vi "Bearing to graph.vi"(10 "Bearing":dbl=0.1) -> (2 "XY Graph":cluster{dbl[], dbl[]}(graph))   [LabVIEW 2009]
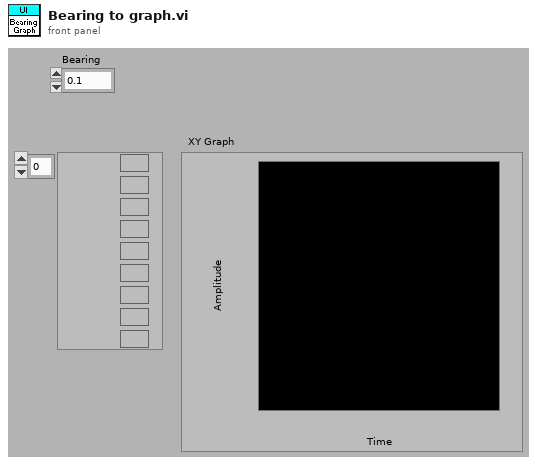
[diagram p1: front panel]
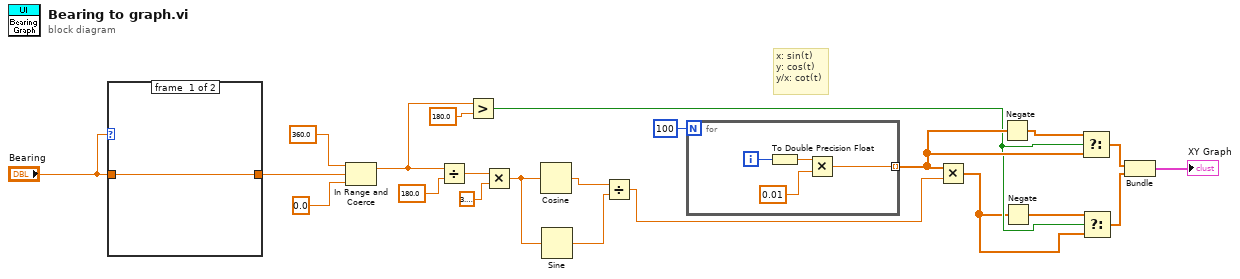
[diagram p0: block diagram]
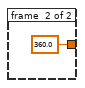
[diagram p2: hidden frame]
diagram:
  # "x: sin(t)\ny: cos(t)\ny/x: cot(t)"
  n1 = case shown="Default" "Bearing" {
    tunnel: [w23 360.0 ("Bearing")] -> w14
    tunnel: "Bearing" -> [w23 _]
    frame #0 {
    }
    frame #1 {
    }
  }
  n2 = In Range and Coerce(upper limit=360.0, x=w14, lower limit=0.0) -> (coerced(x)=w11:dbl)  [unwired: 1 out]
  n3 = Divide(x=w11, y=180.0) -> (x/y=w20:dbl)
  n4 = Greater?(x=w11, y=180.0) -> (0:w5:bool)
  n5 = Multiply(x=w20, y=3.141592653589793) -> (x*y=w18:dbl)
  n6 = Cosine(x=w18) -> (cos(x)=w16:dbl)
  n7 = Sine(x=w18) -> (sin(x)=w15:dbl)
  n8 = Divide(x=w16, y=w15) -> (x/y=w17:dbl)
  n9 = for {
    N: 100 -> [_]
    tunnel: [w25] -> w8 mode=indexing
    i -> [w28]
    n10 = To Double Precision Float(number=w28) -> (double precision float=w27:dbl)
    n11 = Multiply(x=w27, y=0.01) -> (x*y=w25:dbl)
  }
  n12 = Multiply(x=w8, y=w17) -> (x*y=w4:dbl[])
  n13 = Negate(x=w8) -> (-x=w9:dbl[])
  n14 = Negate(x=w4) -> (-x=w6:dbl[])
  n15 = Select(t=w9, s=w5, f=w8) -> (s? t:f=w7:dbl[])
  n16 = Select(t=w6, s=w5, f=w4) -> (s? t:f=w3:dbl[])
  n17 = Bundle(w7, w3) -> (→"XY Graph":cluster{dbl[], dbl[]})  [unwired: 1 in]
